vi "Set Single Digital Out.vi"(6 "Target Digital out":u32, 8 "error in":errorcluster, 10 "Value to Write":bool, 11 "DIG_IO in":refnum<class "DIG_IO.lvclass">) -> (0 "error out":errorcluster, 3 "DIG_IO out":refnum<class "DIG_IO.lvclass">)   [LabVIEW 2019, in "DIG_IO.lvlib" / "DIG_IO.lvclass"]
doc: "Set addressed input to the specified state (ON/OFF) \n\nTarget Digital out is a U32 which is the largest datatype that an enum can be.\nThis is so that the top level test can use a typedefinition enum to define the digital output mapping."
uses:
  Library/DIG_IO.lvclass
  Library/DIG_IO.lvclass/DIG_IO.ctl
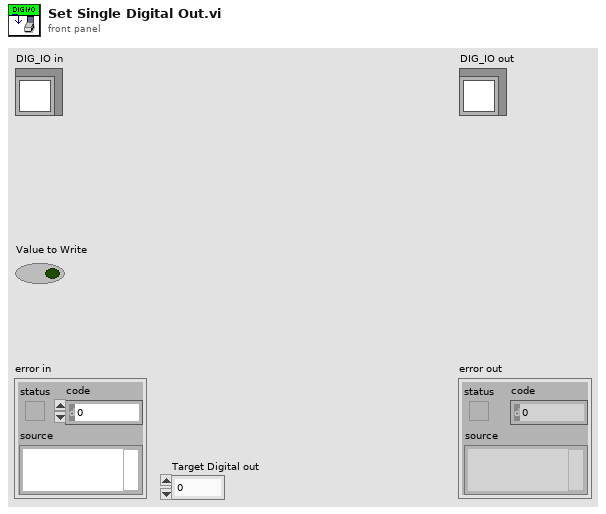
[diagram p1: front panel]
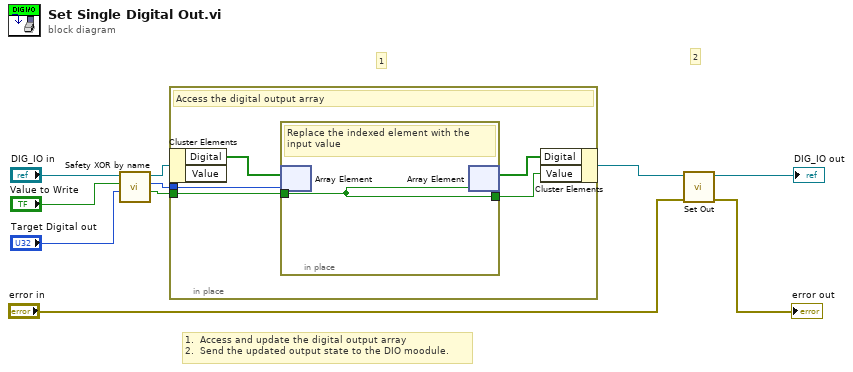
[diagram p0: block diagram]
diagram:
  # "1.  Access and update the digital output array\n2.  Send the updated output state to the DIO moodule."
  # "2"
  # "1"
  n1 = call "Safety XOR by name.vi"("Target Digital in"="Target Digital out", "Value to Write"="Value to Write", "DIG_IO in"="DIG_IO in") -> ("Value Select"=w1:bool, "Target Digital out"=w2:u32, "DIG_IO out"=w5:refnum<class "DIG_IO.lvclass">)  [unwired: 5 in, 1 out]
  n2 = in-place {
    in-place-border: w2 -> [w14]
    in-place-border: w1 -> [w12]
    # "Access the digital output array"
    n3 = in-place-cluster #1(w5) -> ("Digital"=w15:bool[])  [unwired: 1 out]
    n4 = in-place {
      in-place-border: w12 -> [w16]
      in-place-border: [w16] -> w11
      # "Replace the indexed element with the input value"
      n5 = in-place-array #2(w15, w14) -> ()  [unwired: 1 out]
      n6 = in-place-array #2(w16) -> (w13:bool[])  [unwired: 1 out]
    }
    n7 = in-place-cluster #1("Digital"=w13, "Value"=w11) -> (w7:refnum<class "DIG_IO.lvclass">)
  }
  n8 = call-dynamic "Set Out.vi"("error in"="error in", "DIG_IO in"=w7) -> ("error out"=→"error out":errorcluster, "DIG_IO out"=→"DIG_IO out":refnum<class "DIG_IO.lvclass">)  [unwired: 8 in]
